vi "CVT Globals.vi"() -> ()   [LabVIEW 2016, in "CVT.lvlib" / "Current Value Table.lvlib"]
uses:
  Current Value Table.lvlib
panel:
  out "Reset count":u32
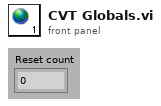
[diagram p1: front panel]
diagram:
